vi "DAQ Loop.vi"(8 "error in (no error)":errorcluster caption="错误输入（无错误）", 9 "数据通知器":refnum<notifier>, 10 "DAQ":refnum<queue>, 11 "Director":refnum<queue>) -> (0 "error out":errorcluster caption="错误输出")   [LabVIEW 2015, in "DAQ.lvlib"]
doc: "该消息循环负责处理硬件数据采集的相关消息。"
uses:
  DAQ.lvlib
  support/Message Queue/Message Cluster.ctl
  DAQ Configuration.ctl
  Support/DAQ State.ctl
  support/Message Queue/Enqueue Message (Single).vi
  <vilib>/Utility/error.llb/Error Cluster From Error Code.vi
  <vilib>/ErrorRing/Error Ring.xnode
  support/Message Queue/Message Queue.lvlib
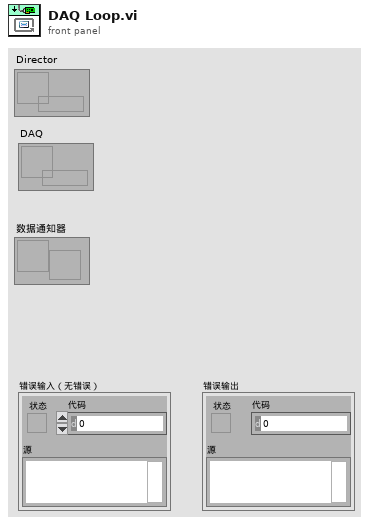
[diagram p1: front panel]
types:
  T1 = typedef "DAQ.lvlib/DAQ State.ctl" = enum16{"Idle", "Acquiring"}
  T2 = typedef "DAQ.lvlib/DAQ Configuration.ctl" = cluster{"hDevice":i32, "DevNum":u8, "Configuration Parameter":i32[], "READ_MAX_LEN":i32, "DO":bool[]}
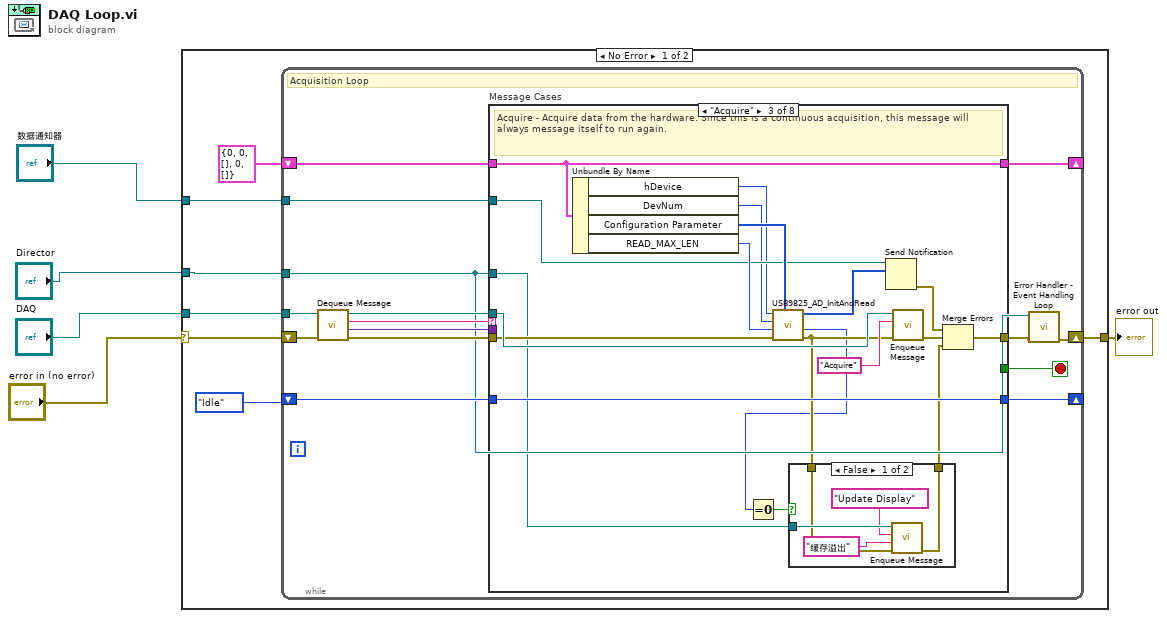
[diagram p0: block diagram]
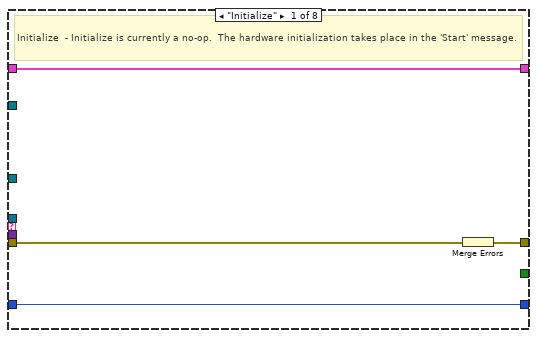
[diagram p2: hidden frame]
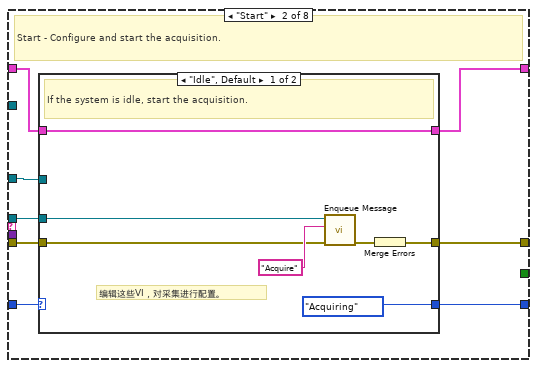
[diagram p3: hidden frame]
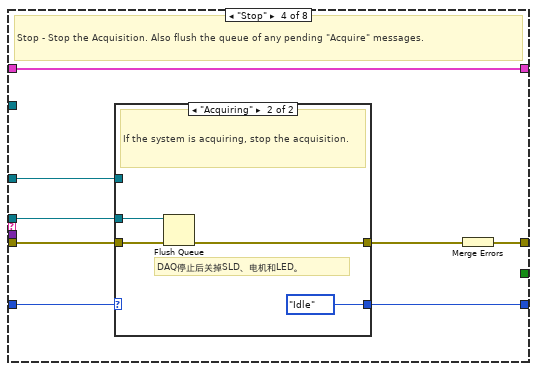
[diagram p6: hidden frame]
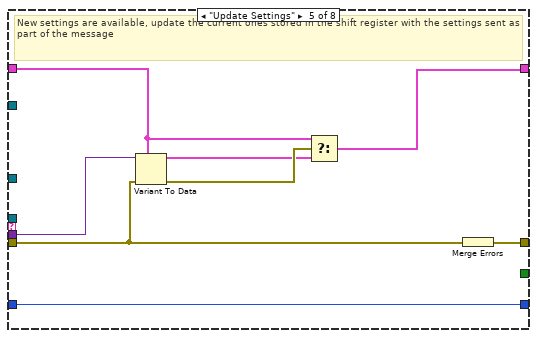
[diagram p8: hidden frame]
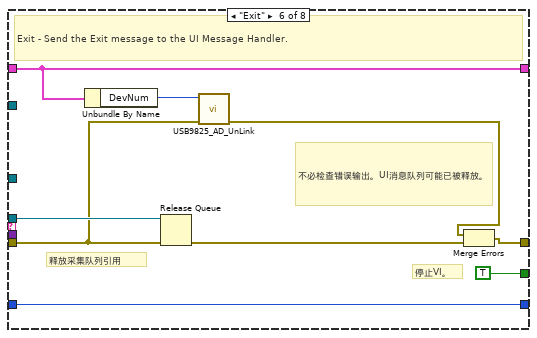
[diagram p9: hidden frame]
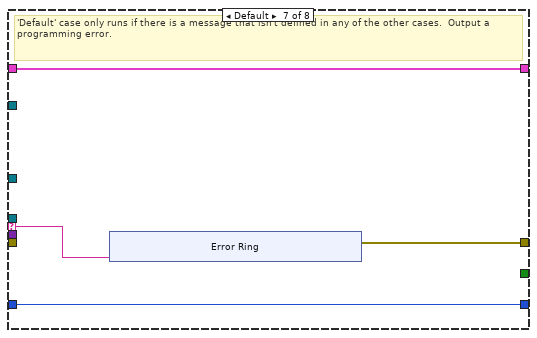
[diagram p10: hidden frame]
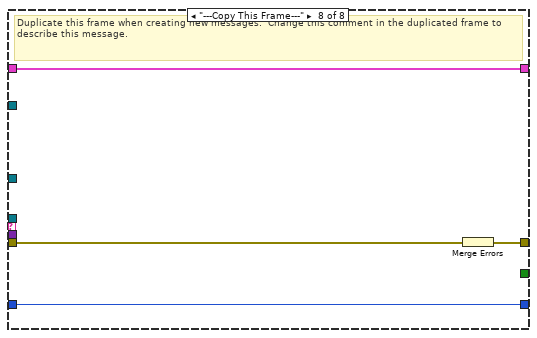
[diagram p11: hidden frame]
diagram:
  n1 = case shown="No Error" "error in (no error)" {
    selector: "error in (no error)" -> [w11 w121]
    tunnel: [w12 w121] -> w5
    tunnel: "数据通知器" -> [w8 _]
    tunnel: "DAQ" -> [w7 _]
    tunnel: "Director" -> [w6 _]
    frame No Error {
      n2 = while {
        tunnel: w7 -> [w19]
        shift-right: [w26] -> _
        shift-left: T2 {"hDevice"=0, "DevNum"=0, "Configuration Parameter"=[], "READ_MAX_LEN"=0, "DO"=[]} ("DAQ Configuration") -> [w27]
        shift-right: [w16] -> w12
        shift-left: w11 -> [w24]
        tunnel: w6 -> [w14]
        shift-right: [w17] -> _
        shift-left: DAQ_State."Idle" ("State") -> [w18]
        tunnel: w8 -> [w13]
        stop <- w25 stop-if-true
        # "Acquisition Loop"
        n3 = call "Dequeue Message.vi"("error in (no error)"=w24, "消息队列"=w19) -> ("error out"=w23:cluster{"状态":bool, "代码":i32, "源":string}, "消息数据"=w21:variant, "消息"=w22:string, "消息队列副本"=w20:refnum<queue>)  [unwired: 6 in]
        n4 = case "Message Cases" shown="\"Acquire\"" w22 {
          selector: w22 -> [_ _ _ _ _ _ w108 _]
          tunnel: w20 -> [_ w36 w66 w79 _ w102 _ _]
          tunnel: w23 -> [w29 w37 w60 w81 w90 w98 _ w120]
          tunnel: [w31 w39 w68 w82 w96 w104 w107 w118] -> w15
          tunnel: w27 -> [w28 w38 w61 w80 w92 w100 w109 w119]
          tunnel: [w28 w35 w61 w80 w91 w100 w109 w119] -> w26
          tunnel: [_ _ _ _ _ TRUE _ _] -> w25
          tunnel: w21 -> [_ _ _ _ w95 _ _ _]
          tunnel: w14 -> [_ w32 w54 w78 _ _ _ _]
          tunnel: w18 -> [w30 w34 w64 w77 w89 w101 w106 w117]
          tunnel: [w30 w33 w64 w76 w89 w101 w106 w117] -> w17
          tunnel: w13 -> [_ _ w59 _ _ _ _ _]
          frame "Initialize" {
            # "Initialize  - Initialize is currently a no-op.  The hardware initialization takes place in the 'Start' message."
            n5 = Merge Errors(w29) -> (w31:errorcluster)
          }
          frame "Start" {
            # "Start - Configure and start the acquisition."
            n6 = case shown="\"Idle\", Default" w34 {
              selector: w34 -> [_ w47]
              tunnel: [w46 w49] -> w39
              tunnel: w38 -> [w40 w48]
              tunnel: w37 -> [w41 w49]
              tunnel: w36 -> [w44 _]
              tunnel: [w40 w48] -> w35
              tunnel: [DAQ_State."Acquiring" ("State") w47] -> w33
              tunnel: w32 -> [_ _]
              frame "Idle", Default {
                # "编辑这些VI，对采集进行配置。"
                # "If the system is idle, start the acquisition."
                n7 = call-poly "Enqueue Message.vi"("error in (no error)"=w41, "消息"="Acquire" ("Message"), "消息队列"=w44) -> ("error out"=w45:cluster{"状态":bool, "代码":i32, "源":string})  [unwired: 7 in, 1 out]
                n8 = Merge Errors(w45) -> (w46:errorcluster)
              }
              frame "Acquiring" {
                # "The system is already acquiring. Ignore the \"Start\" message."
              }
            }
          }
          frame "Acquire" {
            # "Acquire - Acquire data from the hardware. Since this is a continuous acquisition, this message will always message itself to run again."
            n9 = Unbundle By Name(w61) -> ("hDevice"=w56:i32, "DevNum"=w55:u8, "Configuration Parameter"=w63:i32[], "READ_MAX_LEN"=w62:i32)
            n10 = call "USB9825_AD_InitAndRead.vi"("Configuration Parameter"=w63, "错误输入（无错误）"=w60, "READ_MAX_LEN"=w62, "DevNum"=w55, "hDevice"=w56) -> ("错误输出"=w52:errorcluster, "pBufOver"=w50:i32, "AD"=w58:i16[])  [unwired: 3 in, 1 out]
            n11 = Equal To 0?(x=w50) -> (x = 0?=w51:bool)
            n12 = case shown="False" w51 {
              tunnel: w54 -> [w73 _]
              tunnel: [w71 w74] -> w53
              tunnel: w52 -> [w70 w74]
              frame False {
                n13 = call-poly "Enqueue Message.vi"("error in (no error)"=w70, "消息数据"="缓存溢出" ("消息"), "消息"="Update Display", "消息队列"=w73) -> ("error out"=w71:cluster{"状态":bool, "代码":i32, "源":string})  [unwired: 6 in, 1 out]
              }
              frame True {
              }
            }
            n14 = Send Notification(notification=w58, notifier=w59) -> (error out=w57:errorcluster)  [unwired: 1 in, 1 out]
            n15 = call-poly "Enqueue Message.vi"("error in (no error)"=w52, "消息"="Acquire" ("Message"), "消息队列"=w66) -> ("error out"=w67:cluster{"状态":bool, "代码":i32, "源":string})  [unwired: 7 in, 1 out]
            n16 = Merge Errors(w57, w67, w53) -> (w68:errorcluster)
          }
          frame "Stop" {
            # "Stop - Stop the Acquisition. Also flush the queue of any pending \"Acquire\" messages."
            n17 = case shown="\"Acquiring\"" w77 {
              selector: w77 -> [w84 _]
              tunnel: w81 -> [w83 w88]
              tunnel: w79 -> [_ w87]
              tunnel: w78 -> [_ _]
              tunnel: [w84 DAQ_State."Idle" ("State")] -> w76
              tunnel: [w83 w85] -> w75
              frame "Idle", Default {
                # "The system is already idle. Ignore the \"Stop\" message."
              }
              frame "Acquiring" {
                # "DAQ停止后关掉SLD、电机和LED。"
                # "If the system is acquiring, stop the acquisition."
                n18 = Flush Queue(queue=w87, error in (no error)=w88) -> (error out=w85:errorcluster)  [unwired: 2 out]
              }
            }
            n19 = Merge Errors(w75) -> (w82:errorcluster)
          }
          frame "Update Settings" {
            # "New settings are available, update the current ones stored in the shift register with the settings sent as part of the message"
            n20 = Variant To Data(error in=w90, type=w92, Variant=w95) -> (data=w93:T2, error out=w94:errorcluster)
            n21 = Select(t=w92, s=w94, f=w93) -> (s? t:f=w91:T2)
            n22 = Merge Errors(w90) -> (w96:errorcluster)
          }
          frame "Exit" {
            # "不必检查错误输出。UI消息队列可能已被释放。"
            # "释放采集队列引用"
            # "停止VI。"
            # "Exit - Send the Exit message to the UI Message Handler."
            n23 = Unbundle By Name(w100) -> ("DevNum"=w99:u8)
            n24 = Release Queue(queue=w102, error in (no error)=w98) -> (error out=w103:errorcluster)  [unwired: 1 in, 2 out]
            n25 = call "USB9825_AD_UnLink.vi"("Error In"=w98, "hDevice"=w99) -> ("Error Out"=w97:errorcluster)  [unwired: 9 in]
            n26 = Merge Errors(w97, w103) -> (w104:errorcluster)
          }
          frame Default {
            # "'Default' case only runs if there is a message that isn't defined in any of the other cases.  Output a programming error."
            n27 = xnode "Error Ring"("parameter 0"=w108) -> ("error out"=w107:errorcluster)
          }
          frame "---Copy This Frame---" {
            # "Duplicate this frame when creating new messages.  Change this comment in the duplicated frame to describe this message."
            n28 = Merge Errors(w120) -> (w118:errorcluster)
          }
        }
        n29 = call "Error Handler - Event Handling Loop.vi"("error in (no error)"=w15, "消息队列"=w14) -> ("错误输入副本"=w16:cluster{"状态":bool, "代码":i32, "源":string})  [unwired: 8 in, 1 out]
      }
    }
    frame Error {
    }
  }
  "error out" <- w5
